vi "Untitled 1.vi"() -> ()   [LabVIEW 2010]
panel:
  out "elapsed time":dbl[](array[numeric])
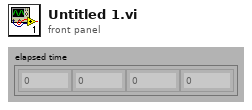
[diagram p1: front panel]
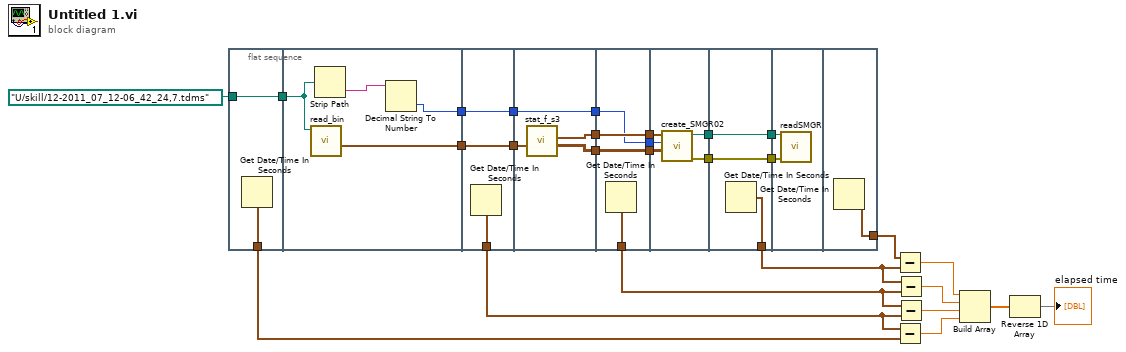
[diagram p0: block diagram]
diagram:
  n1 = flat-sequence {
    tunnel: path "U:/skill/12-2011_07_12-06_42_24,7.tdms" ("datalog path (use dialog)") -> [w29]
    tunnel: [w29] -> w26
    tunnel: [w28] -> w10
    tunnel: w26 -> [w32]
    tunnel: [w30] -> w24
    tunnel: [w31] -> w15
    tunnel: [w36] -> w25
    tunnel: w24 -> [w36]
    tunnel: w15 -> [w35]
    tunnel: [w35] -> w14
    tunnel: [w34] -> w7
    tunnel: w25 -> [w40]
    tunnel: [w39] -> w23
    tunnel: [w38] -> w21
    tunnel: w14 -> [w37]
    tunnel: [w37] -> w13
    tunnel: w23 -> [w44]
    tunnel: [w44] -> w22
    tunnel: w21 -> [w43]
    tunnel: [w43] -> w20
    tunnel: w13 -> [w42]
    tunnel: [w42] -> w12
    tunnel: [w41] -> w8
    tunnel: w22 -> [w49]
    tunnel: w20 -> [w48]
    tunnel: [w47] -> w18
    tunnel: [w46] -> w16
    tunnel: w12 -> [w45]
    tunnel: [w52] -> w19
    tunnel: w18 -> [w52]
    tunnel: [w51] -> w17
    tunnel: w16 -> [w51]
    tunnel: [w50] -> w9
    tunnel: w19 -> [w54]
    tunnel: w17 -> [w53]
    tunnel: [w55] -> w11
    frame #0 {
      n2 = Get Date/Time In Seconds() -> (seconds since 1Jan1904=w28:timestamp)
    }
    frame #1 {
      n3 = call "read_bin.vi"("datalog path (use dialog)"=w32) -> ("Waveform Graph"=w30:waveform(i16)[])  [unwired: 4 in, 2 out]
      n4 = Strip Path(path=w32) -> (name=w33:string)  [unwired: 1 out]
      n5 = Decimal String To Number(string=w33) -> (number=w31:i32)  [unwired: 2 in, 1 out]
    }
    frame #2 {
      n6 = Get Date/Time In Seconds() -> (seconds since 1Jan1904=w34:timestamp)
    }
    frame #3 {
      n7 = call "stat_f_s3.vi"("Array of Waveform"=w40) -> ("Array 2"=w38:waveform(i16)[][], "sync"=w39:waveform(i16))  [unwired: 5 in]
    }
    frame #4 {
      n8 = Get Date/Time In Seconds() -> (seconds since 1Jan1904=w41:timestamp)
    }
    frame #5 {
      n9 = call "create_SMGR02.vi"("array"=w48, "meas_point"=w45, "sync"=w49) -> ("error out"=w46:errorcluster, "path"=w47:path)  [unwired: 3 in]
    }
    frame #6 {
      n10 = Get Date/Time In Seconds() -> (seconds since 1Jan1904=w50:timestamp)
    }
    frame #7 {
      n11 = call "readSMGR.vi"("error in"=w53, "file path"=w54) -> ()  [unwired: 3 in, 3 out]
    }
    frame #8 {
      n12 = Get Date/Time In Seconds() -> (seconds since 1Jan1904=w55:timestamp)
    }
  }
  n13 = Subtract(x=w11, y=w9) -> (x-y=w6:dbl)
  n14 = Subtract(x=w7, y=w10) -> (x-y=w3:dbl)
  n15 = Subtract(x=w9, y=w8) -> (x-y=w5:dbl)
  n16 = Subtract(x=w8, y=w7) -> (x-y=w4:dbl)
  n17 = Build Array(w6, w5, w4, w3) -> (w2:dbl[])
  n18 = Reverse 1D Array(array=w2) -> (reversed array=→"elapsed time":dbl[])
